vi "Build Spec System Explorer.vi"(9 "Action":T1) -> (1 "Output":string)   [LabVIEW 2019, in "NIVS_Consolidated_CDW_MetaDataObj.lvclass"]
doc: "Constants, which are necessary for the <B>CD System Explorer LLB</B> in the generated custom device."
uses:
  NIVS_Consolidated_CDW_MetaDataObj.lvclass
  Build Spec System Explorer.ctl
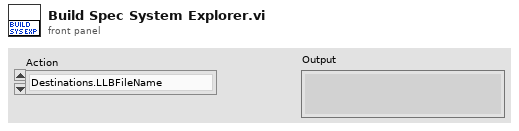
[diagram p1: front panel]
types:
  T1 = typedef "NIVS_Consolidated_CDW_MetaDataObj.lvclass/Build Spec System Explorer.ctl" = enum16{"Destinations.LLBFileName"}
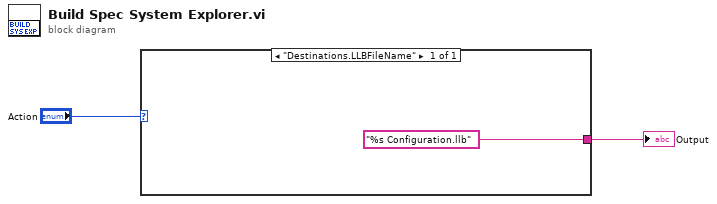
[diagram p0: block diagram]
diagram:
  n1 = case shown="\"Destinations.LLBFileName\"" "Action" {
    tunnel: ["%s Configuration.llb"] -> w1
    frame "Destinations.LLBFileName" {
    }
  }
  "Output" <- w1
